vi "Stop Work.vi"(6 "Controller name":string, 8 "error in (no error)":errorcluster, 9 "Reply":bool=TRUE, 10 "Reply to":refnum<class "Stop Response Msg.lvclass">, 11 "Measure Object in":refnum<class "Lockin Digitizer.lvclass">) -> (0 "error out":errorcluster, 3 "Measure Object out":refnum<class "Lockin Digitizer.lvclass">)   [LabVIEW 2021, in "Lockin Digitizer.lvclass"]
uses:
  Lockin Digitizer.lvclass
  Controllers/Process Controller Messages/Stop Response Msg/Stop Response Msg.lvclass
  Lockin Digitizer.lvclass/Lockin Digitizer.ctl
  Pulse Recorder Actor/Pulse Recorder Actor.lvclass
  NHMFL_Core/Libraries/Instruments/Instrument Driver/Worker State.ctl
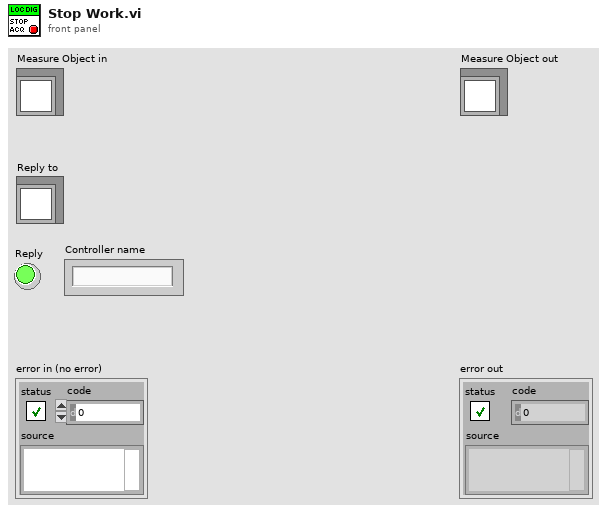
[diagram p1: front panel]
types:
  T1 = typedef "Worker State.ctl" = enum16{"Idle", "Starting", "Working", "Stopping"}
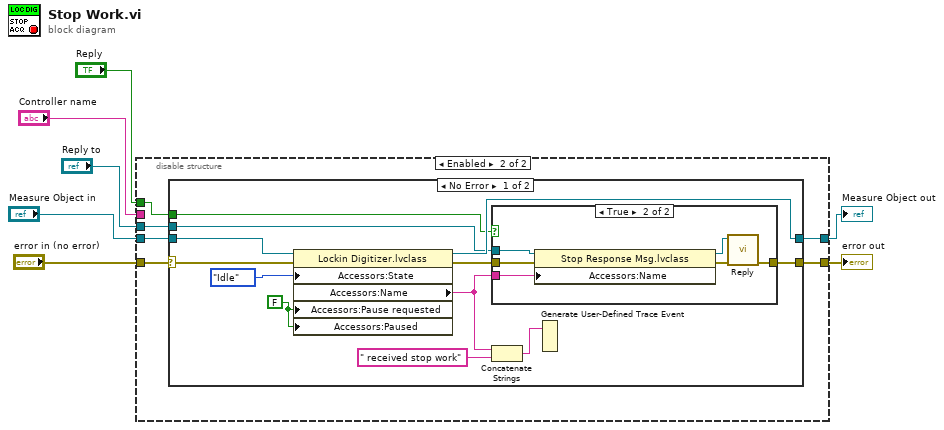
[diagram p0: block diagram]
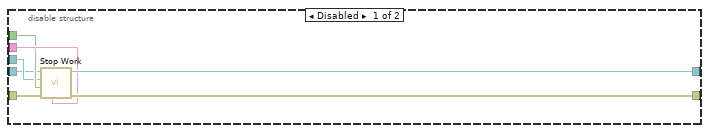
[diagram p2: hidden frame]
diagram:
  n1 = disable-structure shown="Enabled" {
    disable-tunnel: [w14 w18] -> w7
    disable-tunnel: [w13 w15] -> w6
    disable-tunnel: "Controller name" -> [w12 _]
    disable-tunnel: "error in (no error)" -> [w11 w17]
    disable-tunnel: "Reply" -> [w10 w16]
    disable-tunnel: "Reply to" -> [w9 w19]
    disable-tunnel: "Measure Object in" -> [w8 w20]
    frame Disabled {
      n2 = call-parent "Stop Work.vi"("Controller name"=w12, "error in (no error)"=w11, "Reply"=w10, "Reply to"=w9, "Measure Object in"=w8) -> ("error out"=w14:errorcluster, "Measure Object out"=w13:refnum<class "Lockin Digitizer.lvclass">)  [unwired: 5 in]
    }
    frame Enabled {
      n3 = case shown="No Error" w17 {
        selector: w17 -> [w30 w41]
        tunnel: [w23 w41] -> w18
        tunnel: [w31 w40] -> w15
        tunnel: w20 -> [w32 w40]
        tunnel: w19 -> [w26 _]
        tunnel: w16 -> [w22 _]
        frame No Error {
          w21 = FALSE ("Pause requested")
          n4 = property class="Lockin Digitizer.lvclass"(reference=w32, error in=w30, "Accessors:State"=Worker_State."Idle" ("State"), "Accessors:Pause requested"=w21, "Accessors:Paused"=w21) -> (reference out=w31:refnum<class "Lockin Digitizer.lvclass">, error out=w24:errorcluster, "Accessors:Name"=w25:string)
          n5 = case shown="True" w22 {
            tunnel: w26 -> [_ w39]
            tunnel: w25 -> [_ w38]
            tunnel: w24 -> [w33 w37]
            tunnel: [w33 w34] -> w23
            frame False {
            }
            frame True {
              n6 = property class="Stop Response Msg.lvclass"(reference=w39, error in=w37, "Accessors:Name"=w38) -> (reference out=w36:refnum<class "Stop Response Msg.lvclass">, error out=w35:errorcluster)
              n7 = call-dynamic "Reply.vi"("error in (no error)"=w35, "Self-addressed Msg in"=w36) -> ("error out"=w34:errorcluster)  [unwired: 8 in, 1 out]
            }
          }
          n8 = Concatenate Strings(w25, " received stop work" ("string")) -> (w28:string)
          n9 = Generate User-Defined Trace Event(2:w28) -> ()  [unwired: 1 in]
        }
        frame Error {
        }
      }
    }
  }
  "error out" <- w7
  "Measure Object out" <- w6
